vi "Update Limit Values.vi"(0 "Limits I1":cluster{"Lower":dbl, "Upper":dbl, "Actual":dbl}, 1 "Limits I2":cluster{"Lower":dbl, "Upper":dbl, "Actual":dbl}, 2 "Limits I3":cluster{"Lower":dbl, "Upper":dbl, "Actual":dbl}, 3 "Limits  I4":cluster{"Lower":dbl, "Upper":dbl, "Actual":dbl}, 4 "Limits I5":cluster{"Lower":dbl, "Upper":dbl, "Actual":dbl}, 5 "Limits I6":cluster{"Lower":dbl, "Upper":dbl, "Actual":dbl}, 6 "Data":dbl[](array[numeric]), 8 "Value Slot":T1) -> (14 "Limits O1":cluster{"Lower":dbl, "Upper":dbl, "Actual":dbl}, 15 "Limits O2":cluster{"Lower":dbl, "Upper":dbl, "Actual":dbl}, 16 "Limits O3":cluster{"Lower":dbl, "Upper":dbl, "Actual":dbl}, 17 "Limits  O4":cluster{"Lower":dbl, "Upper":dbl, "Actual":dbl}, 18 "Limits O5":cluster{"Lower":dbl, "Upper":dbl, "Actual":dbl}, 19 "Limits O6":cluster{"Lower":dbl, "Upper":dbl, "Actual":dbl})   [LabVIEW 2013]
uses:
  Value Slot.ctl
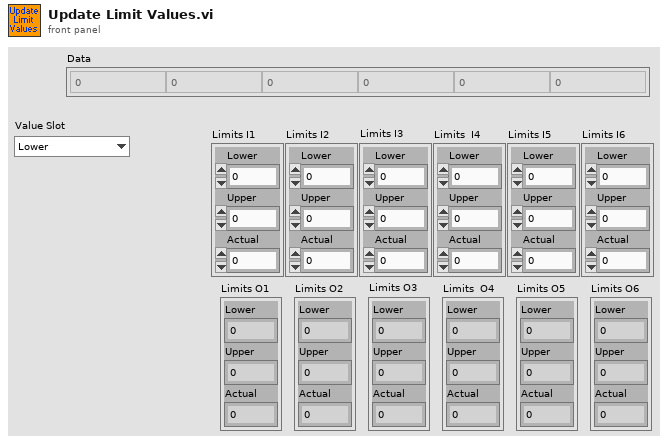
[diagram p1: front panel]
types:
  T1 = typedef "Value Slot.ctl" = enum16{"Lower", "Upper", "Actual"}
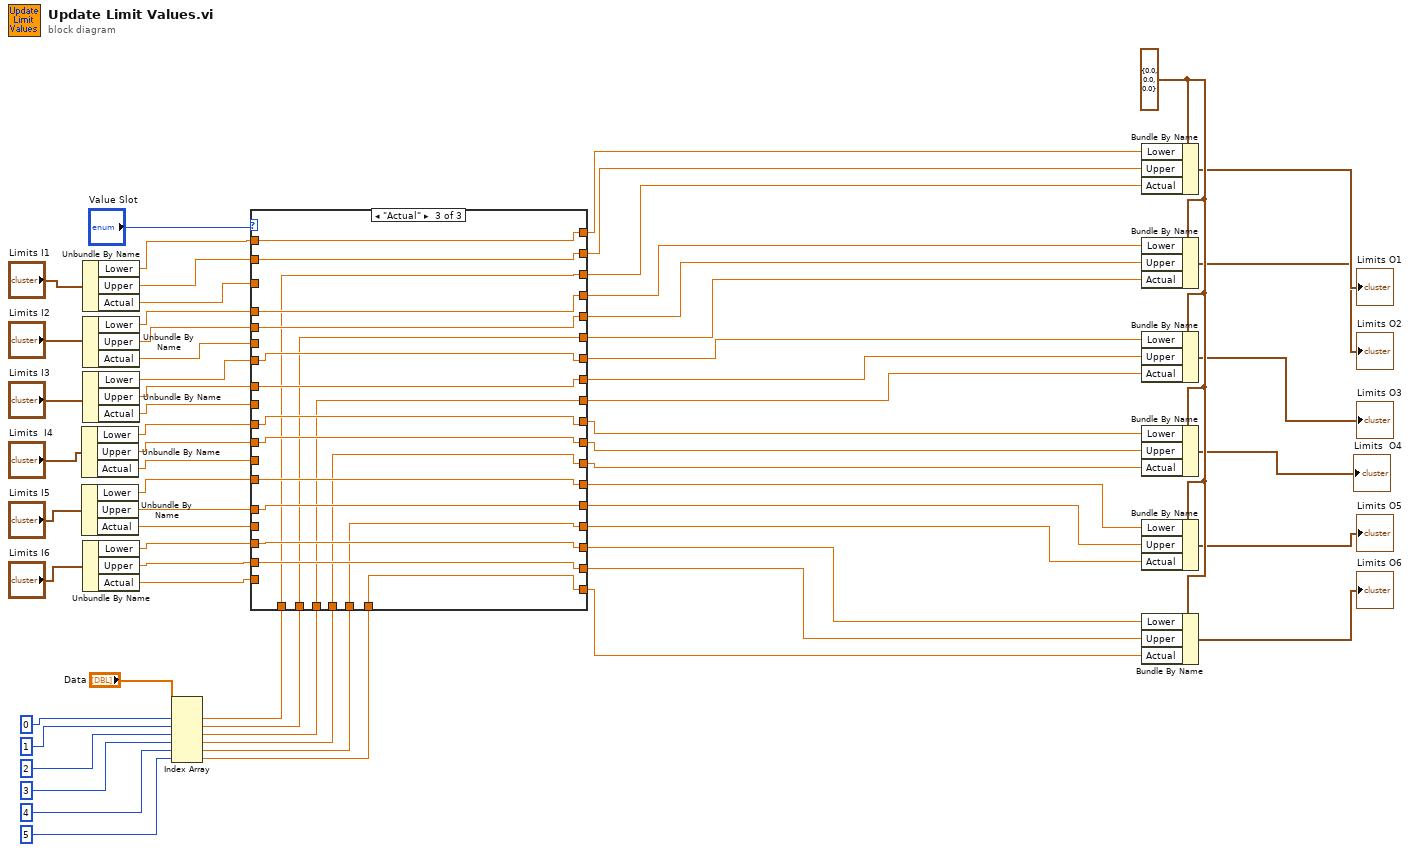
[diagram p0: block diagram]
diagram:
  w63 = cluster{"Lower":dbl, "Upper":dbl, "Actual":dbl} {"Lower"=0.0, "Upper"=0.0, "Actual"=0.0} ("Limits X 5")
  n1 = Unbundle By Name("Limits  I4") -> ("Lower"=w22:dbl, "Upper"=w21:dbl, "Actual"=w20:dbl)
  n2 = Unbundle By Name("Limits I5") -> ("Lower"=w19:dbl, "Upper"=w18:dbl, "Actual"=w17:dbl)
  n3 = Unbundle By Name("Limits I1") -> ("Lower"=w31:dbl, "Upper"=w30:dbl, "Actual"=w29:dbl)
  n4 = Unbundle By Name("Limits I2") -> ("Lower"=w28:dbl, "Upper"=w27:dbl, "Actual"=w26:dbl)
  n5 = Unbundle By Name("Limits I3") -> ("Lower"=w25:dbl, "Upper"=w24:dbl, "Actual"=w23:dbl)
  n6 = Unbundle By Name("Limits I6") -> ("Lower"=w16:dbl, "Upper"=w15:dbl, "Actual"=w14:dbl)
  n7 = Index Array(array="Data", index #1=0 ("index"), index #2=1 ("index"), index #3=2 ("index"), index #4=3 ("index"), index #5=4 ("index"), index #6=5 ("index")) -> (element #1=w6:dbl, element #2=w5:dbl, element #3=w4:dbl, element #4=w3:dbl, element #5=w2:dbl, element #6=w1:dbl)
  n8 = case shown="\"Actual\"" "Value Slot" {
    tunnel: [w70 w82 w106] -> w62
    tunnel: [w64 w88 w112] -> w61
    tunnel: [w73 w83 w107] -> w60
    tunnel: [w65 w89 w113] -> w59
    tunnel: [w75 w84 w108] -> w58
    tunnel: [w66 w90 w114] -> w57
    tunnel: [w77 w85 w109] -> w56
    tunnel: [w67 w91 w115] -> w55
    tunnel: [w79 w86 w110] -> w54
    tunnel: [w68 w92 w116] -> w53
    tunnel: [w81 w87 w111] -> w52
    tunnel: [w69 w93 w117] -> w51
    tunnel: [w80 w99 w105] -> w43
    tunnel: [w78 w98 w104] -> w42
    tunnel: [w76 w97 w103] -> w41
    tunnel: [w74 w96 w102] -> w40
    tunnel: [w72 w95 w101] -> w39
    tunnel: [w71 w94 w100] -> w38
    tunnel: w31 -> [_ w93 w117]
    tunnel: w30 -> [w81 _ w111]
    tunnel: w29 -> [w80 w99 _]
    tunnel: w28 -> [_ w92 w116]
    tunnel: w27 -> [w79 _ w110]
    tunnel: w26 -> [w78 w98 _]
    tunnel: w25 -> [_ w91 w115]
    tunnel: w24 -> [w77 _ w109]
    tunnel: w23 -> [w76 w97 _]
    tunnel: w22 -> [_ w90 w114]
    tunnel: w21 -> [w75 _ w108]
    tunnel: w20 -> [w74 w96 _]
    tunnel: w19 -> [_ w89 w113]
    tunnel: w18 -> [w73 _ w107]
    tunnel: w17 -> [w72 w95 _]
    tunnel: w16 -> [_ w88 w112]
    tunnel: w15 -> [w70 _ w106]
    tunnel: w14 -> [w71 w94 _]
    tunnel: w6 -> [w69 w87 w105]
    tunnel: w5 -> [w68 w86 w104]
    tunnel: w4 -> [w67 w85 w103]
    tunnel: w3 -> [w66 w84 w102]
    tunnel: w2 -> [w65 w83 w101]
    tunnel: w1 -> [w64 w82 w100]
    frame "Lower" {
    }
    frame "Upper" {
    }
    frame "Actual" {
    }
  }
  n9 = Bundle By Name(cluster=w63, "Lower"=w51, "Upper"=w52, "Actual"=w43) -> (→"Limits O1":cluster{"Lower":dbl, "Upper":dbl, "Actual":dbl})
  n10 = Bundle By Name(cluster=w63, "Lower"=w53, "Upper"=w54, "Actual"=w42) -> (→"Limits O2":cluster{"Lower":dbl, "Upper":dbl, "Actual":dbl})
  n11 = Bundle By Name(cluster=w63, "Lower"=w55, "Upper"=w56, "Actual"=w41) -> (→"Limits O3":cluster{"Lower":dbl, "Upper":dbl, "Actual":dbl})
  n12 = Bundle By Name(cluster=w63, "Lower"=w57, "Upper"=w58, "Actual"=w40) -> (→"Limits  O4":cluster{"Lower":dbl, "Upper":dbl, "Actual":dbl})
  n13 = Bundle By Name(cluster=w63, "Lower"=w59, "Upper"=w60, "Actual"=w39) -> (→"Limits O5":cluster{"Lower":dbl, "Upper":dbl, "Actual":dbl})
  n14 = Bundle By Name(cluster=w63, "Lower"=w61, "Upper"=w62, "Actual"=w38) -> (→"Limits O6":cluster{"Lower":dbl, "Upper":dbl, "Actual":dbl})
